vi "LS_372_set_zone_properties_variabel_ramprate.vi"(11 "Ramprate":dbl) -> ()   [LabVIEW 2019]
uses:
  Global/Global Variables/Data_Display_global.vi
  Instrument_Setup.vi
  Equipment/Lake Shore 372/Lake Shore 372.lvlib
panel:
  out "Pfad zu Heater Table highT":path
  out "Pfad zu Heater Table Low T":path
  out "HeaterZone Tuning Table.txt":string caption="PID Table"
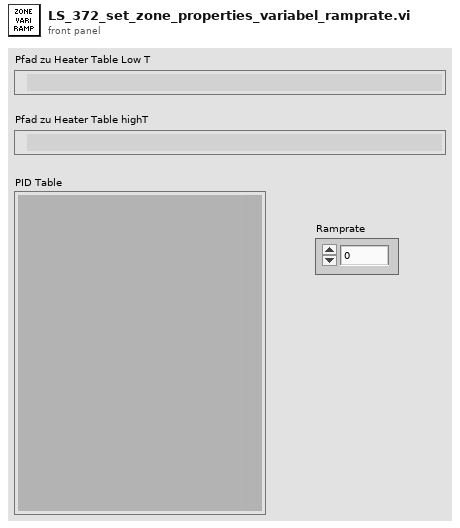
[diagram p1: front panel]
types:
  T1 = enum16{"open", "replace", "create", "open or create", "replace or create", "replace or create with confirmation"}
  T2 = typedef "LS372-Cluster.ctl" = cluster{"Activate Tsweep":bool, "Setpoint - Manual":dbl, "Rate (K/min)":dbl, "Update Lakeshores":bool, "Still Heater":bool, "Still Power (mW)":dbl, "Manual Heater":bool, "Manual Heater  (mW) ":dbl, "Heater Range":dbl, "P (Gain)":dbl, "I (Reset)":dbl, "D (Rate)":dbl, "Heater Power (mW)":dbl, "MC Thermometer":u16, "MC Temperature":dbl, "LS372-T1":dbl, "LS372 -T2":dbl, "LS372-R1 ":dbl, "LS372-R2":dbl, "LS372-T3":dbl, "LS372-T4":dbl, "LS372-R3 ":dbl, "LS372-R4 \n\n\n\n":dbl, "LS372-T5":dbl, "LS372-T6":dbl, "LS372-R5":dbl, "LS372-R6 ":dbl, "Still Power ist":dbl, "Set Temperatur Sweep main":bool, "Setpoint ist":dbl, "Disable Heater":bool}
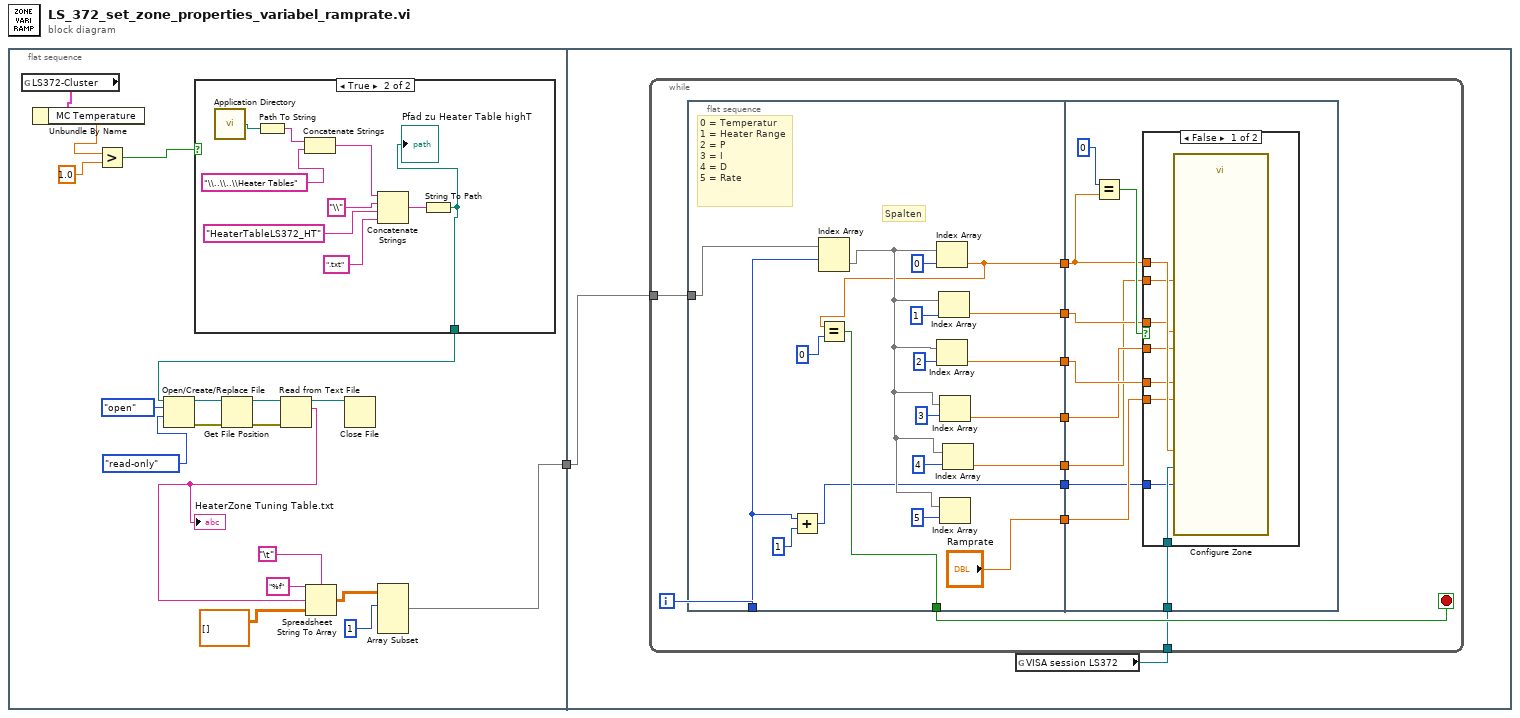
[diagram p0: block diagram]
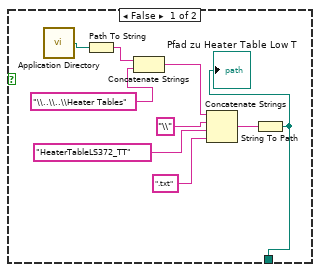
[diagram p2: hidden frame]
diagram:
  n1 = flat-sequence {
    tunnel: [w7] -> w1
    tunnel: w1 -> [w40]
    frame #0 {
      n2 = global read "Data_Display_global.vi" "LS372-Cluster"() -> (w6:T2)
      n3 = Unbundle By Name(w6) -> ("MC Temperature"=w5:dbl)
      n4 = Greater?(x=w5, y=1.0) -> (0:w3:bool)
      n5 = case shown="True" w3 {
        tunnel: [w21 w30] -> w2
        frame False {
          n6 = call <vilib>:"Application Directory.vi"() -> ("Application Directory"=w29:path)
          n7 = Path To String(path=w29) -> (string=w28:string)
          n8 = Concatenate Strings(w28, "\\..\\..\\Heater Tables") -> (w26:string)
          n9 = Concatenate Strings(w26, "\\", "HeaterTableLS372_TT", ".txt") -> (w22:string)
          n10 = String To Path(string=w22) -> (path=w21:path)
          "Pfad zu Heater Table Low T" <- w21
        }
        frame True {
          n11 = call <vilib>:"Application Directory.vi"() -> ("Application Directory"=w38:path)
          n12 = Path To String(path=w38) -> (string=w37:string)
          n13 = Concatenate Strings(w37, "\\..\\..\\Heater Tables") -> (w35:string)
          n14 = Concatenate Strings(w35, "\\", "HeaterTableLS372_HT", ".txt") -> (w31:string)
          n15 = String To Path(string=w31) -> (path=w30:path)
          "Pfad zu Heater Table highT" <- w30
        }
      }
      n16 = Open/Create/Replace File(file path (use dialog)=w2, operation (0:open)=T1."open", access (0:read/write)=enum16{"read/write", "read-only", "write-only"}."read-only") -> (refnum out=w19:refnum<file>, error out=w20:errorcluster)  [unwired: 3 in, 1 out]
      n17 = Get File Position(4:w20, 7:w19) -> (0:w18:errorcluster, 3:w17:refnum<file>)  [unwired: 1 out]
      n18 = Read from Text File(file (use dialog)=w17, error in=w18) -> (refnum out=w16:refnum<file>, text=w11:string)  [unwired: 2 in, 2 out]
      "HeaterZone Tuning Table.txt" <- w11
      n19 = Spreadsheet String To Array(delimiter (Tab)="\t", format string="%f", spreadsheet string=w11, array type (2D Dbl)=dbl[][] []) -> (array=w9:dbl[][])
      n20 = Close File(refnum=w16) -> ()  [unwired: 1 in, 2 out]
      n21 = Array Subset(array=w9, index (row)=1) -> (w7:dbl[][])  [unwired: 3 in]
    }
    frame #1 {
      n22 = global read "Instrument_Setup.vi" "VISA session LS372"() -> (w39:refnum<visa-resource-name>)
      n23 = while {
        tunnel: w40 -> [w51]
        tunnel: w39 -> [w42]
        i -> [w50]
        stop <- w49 stop-if-true
        n24 = flat-sequence {
          tunnel: w51 -> [w70]
          tunnel: w50 -> [w54]
          tunnel: [w60] -> w49
          tunnel: [w62] -> w48
          tunnel: [w59] -> w47
          tunnel: [w58] -> w46
          tunnel: [w57] -> w45
          tunnel: [w56] -> w44
          tunnel: ["Ramprate"] -> w43
          tunnel: [w52] -> w41
          tunnel: w48 -> [w78]
          tunnel: w47 -> [w77]
          tunnel: w46 -> [w76]
          tunnel: w45 -> [w75]
          tunnel: w44 -> [w74]
          tunnel: w43 -> [w73]
          tunnel: w42 -> [w72]
          tunnel: w41 -> [w71]
          frame #0 {
            # "0 = Temperatur\n1 = Heater Range\n2 = P\n3 = I\n4 = D\n5 = Rate"
            # "Spalten"
            n25 = Add(x=w54, y=1) -> (x+y=w52:i32)
            n26 = Index Array(array=w70, index (row)=w54) -> (element=w63:dbl[])  [unwired: 1 in]
            n27 = Index Array(array=w63, index=0) -> (element=w62:dbl)
            n28 = Equal?(x=w62, y=0) -> (x = y?=w60:bool)
            n29 = Index Array(array=w63, index=2) -> (element=w58:dbl)
            n30 = Index Array(array=w63, index=1) -> (element=w59:dbl)
            n31 = Index Array(array=w63, index=3) -> (element=w57:dbl)
            n32 = Index Array(array=w63, index=5) -> ()  [unwired: 1 out]
            n33 = Index Array(array=w63, index=4) -> (element=w56:dbl)
          }
          frame #1 {
            n34 = Equal?(x=0, y=w78) -> (x = y?=w79:bool)
            n35 = case shown="False" w79 {
              tunnel: w78 -> [w88 _]
              tunnel: w77 -> [w87 _]
              tunnel: w76 -> [w86 _]
              tunnel: w75 -> [w85 _]
              tunnel: w74 -> [w84 _]
              tunnel: w73 -> [w83 _]
              tunnel: w72 -> [w82 _]
              tunnel: w71 -> [w81 _]
              frame False {
                n36 = call "Configure Zone.vi"("VISA resource name"=w82, "Zone (1)"=w81, "Upper Bound (0.00000E+0)"=w88, "P Value (10.000)"=w86, "Heater Range (0: Off)"=w87, "I Value (20)"=w85, "Ramp Rate (0)"=w83, "D Value (0)"=w84) -> ()  [unwired: 10 in, 2 out]
              }
              frame True {
              }
            }
          }
        }
      }
    }
  }
